vi "TempControllerMain.vi"() -> ()   [LabVIEW 2013]
uses:
  Controls/stateEnum.ctl
panel:
  in  "Log Folder Location":path=path "E:/USB/LabView/TemperatureController/Data"
  out "Temperature (K)":dbl(graph)
  out "Current Temperature (simulated)":dbl
  out "Current Task":T1
  out "Current Temperature (real)":dbl
  out "Heating up":bool
  in  "Set Point (Max)":dbl
  in  "Monitor\nTemp":bool
  in  "Mode":bool
  in  "Calibrate":bool
  out "Room Temperature (K)":dbl
  out "Resistance @ Room Temperature (ohms)":dbl
  in  "stop":bool
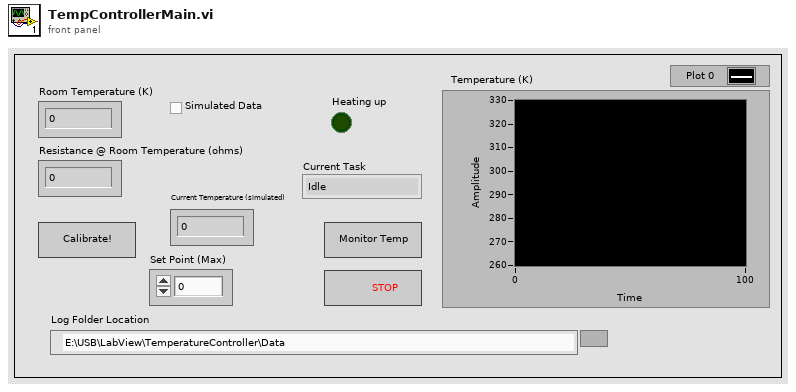
[diagram p1: front panel]
types:
  T1 = typedef "stateEnum.ctl" = enum16{"Idle", "Calibrate", "Initialise", "Set Voltage On", "Set Voltage Off", "Exit"}
  T2 = enum16{"open", "open or create", "create or replace", "create", "open (read-only)"}
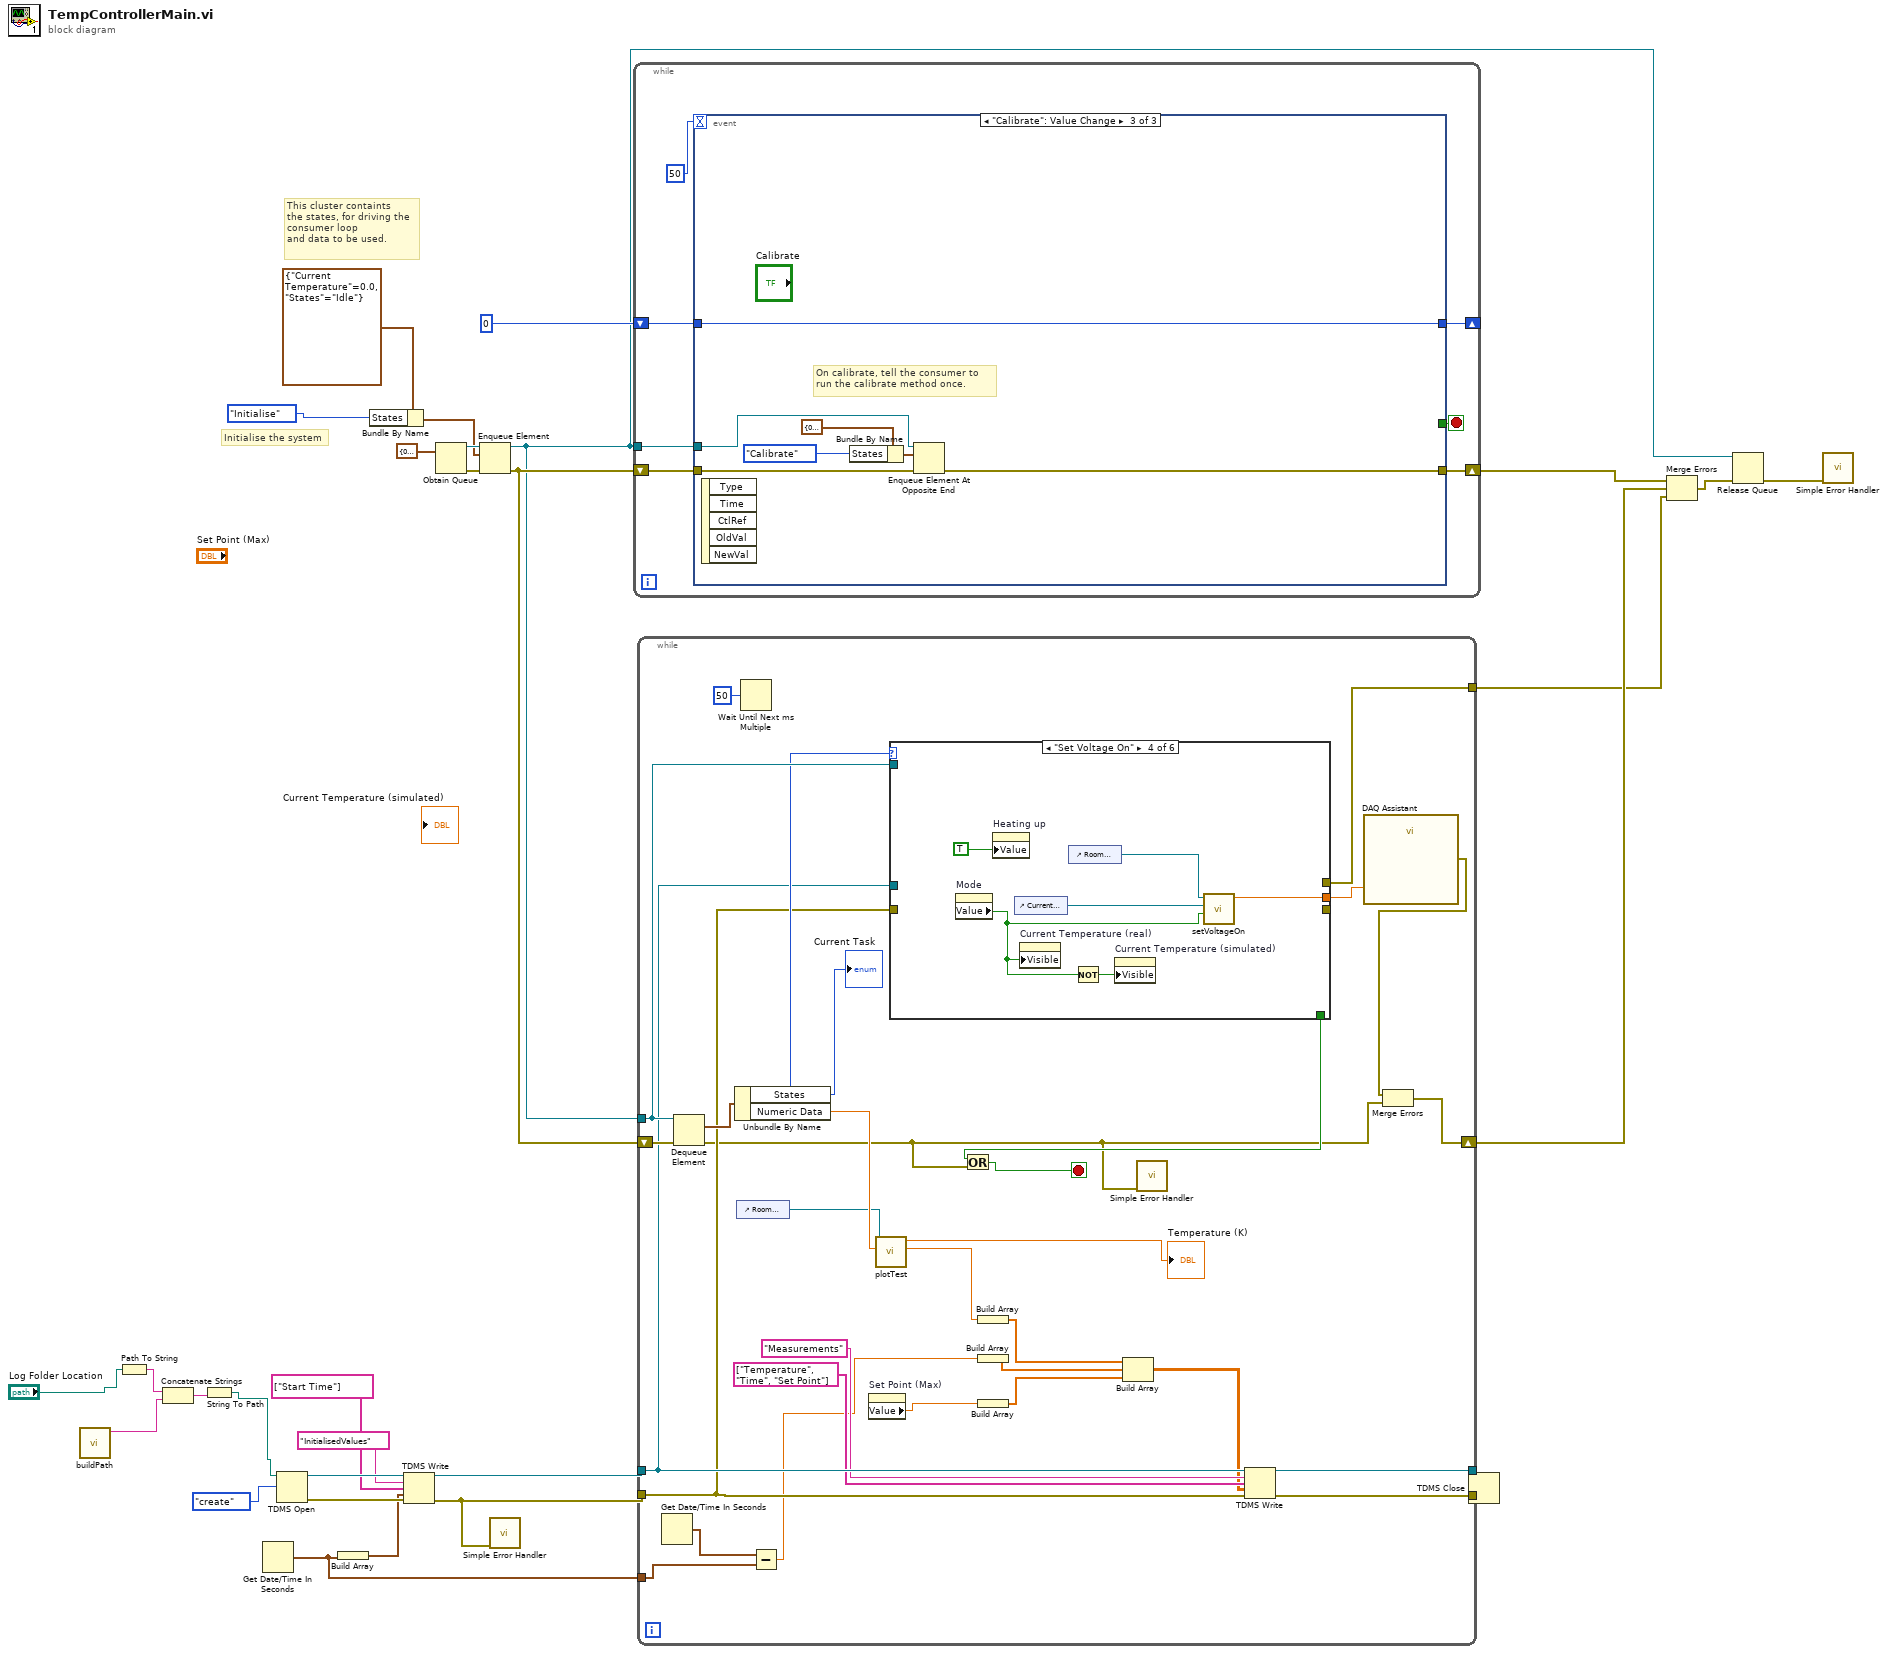
[diagram p0: block diagram]
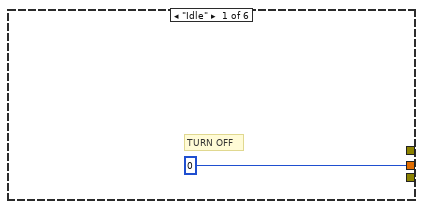
[diagram p2: hidden frame]
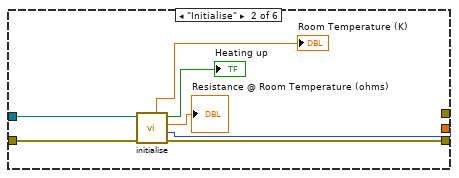
[diagram p3: hidden frame]
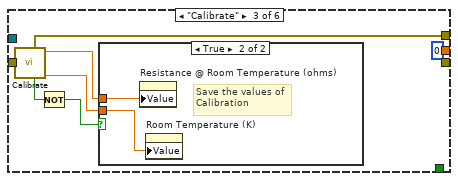
[diagram p4: hidden frame]
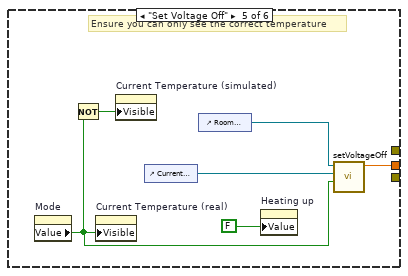
[diagram p6: hidden frame]
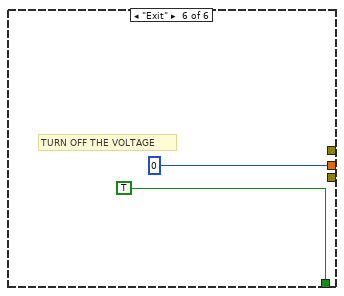
[diagram p7: hidden frame]
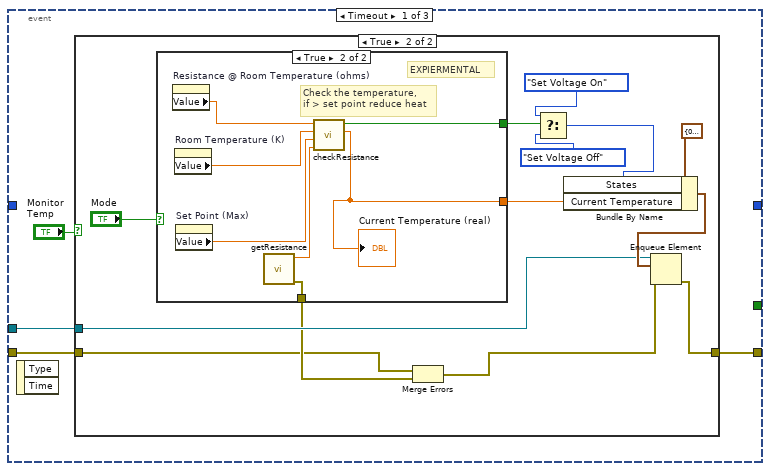
[diagram p8: hidden frame]
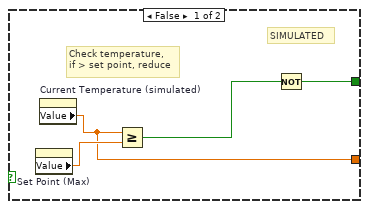
[diagram p10: hidden frame]
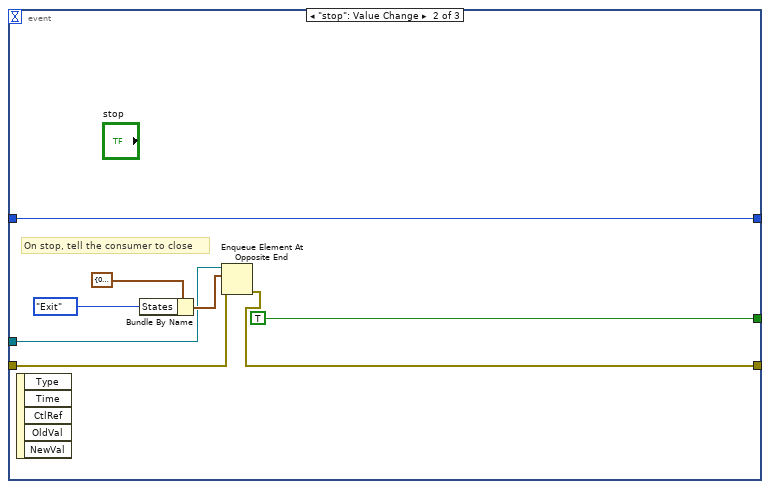
[diagram p11: hidden frame]
diagram:
  # "Initialise the system"
  # "This cluster containts\nthe states, for driving the\nconsumer loop\nand data to be used."
  n1 = call "buildPath.vi"() -> ("String"=w3:string)  [unwired: 11 in]
  n2 = Path To String(path="Log Folder Location") -> (string=w4:string)
  n3 = Concatenate Strings(w4, w3) -> (w2:string)
  n4 = String To Path(string=w2) -> (path=w1:path)
  n5 = Get Date/Time In Seconds() -> (seconds since 1Jan1904=w7:timestamp)
  n6 = TDMS Open(10:T2."create" ("operation (0:open)"), 11:w1) -> (0:w11:errorcluster, 3:w13:refnum<k34>)  [unwired: 5 in]
  n7 = Build Array(w7) -> (w8:timestamp[])
  n8 = Bundle By Name(cluster=cluster{"Current Temperature":dbl, "States":T1} {"Current Temperature"=0.0, "States"=enum."Idle"}, "States"=stateEnum."Initialise") -> (w25:cluster{"Current Temperature":dbl, "States":T1})
  n9 = TDMS Write(0:w13, 5:"InitialisedValues" ("group name in (Untitled)"), 7:string[] ["Start Time"] ("channel name(s) in (Untitled)"), 9:w8, 11:w11) -> (4:w12:refnum<k34>, 15:w6:errorcluster)  [unwired: 1 in, 2 out]
  n10 = Obtain Queue(element data type=cluster{"Numeric Data":dbl, "States":T1} {"Numeric Data"=0.0, "States"=enum."Idle"}) -> (queue out=w29:refnum<queue>, error out=w28:errorcluster)  [unwired: 4 in, 1 out]
  n11 = Enqueue Element(queue=w29, element=w25, error in (no error)=w28) -> (queue out=w19:refnum<queue>, error out=w27:errorcluster)  [unwired: 1 in, 1 out]
  n12 = call <vilib>:"Simple Error Handler.vi"("error in (no error)"=w6) -> ()  [unwired: 4 in, 5 out]
  n13 = while {
    tunnel: w19 -> [w37]
    shift-right: [w34] -> w21
    shift-left: w27 -> [w36]
    shift-right: [w31] -> _
    shift-left: 0 -> [w32]
    stop <- w35 stop-if-true
    n14 = event shown="[2] \"Calibrate\": Value Change" {
      selector: _ -> [_ _ _]
      dyn-events: _ -> [_ _ _]
      timeout: 50 -> [_ _ _]
      tunnel: w37 -> [w41 w69 w80]
      tunnel: w36 -> [w40 w68 w79]
      tunnel: [w38 w67 w78] -> w34
      tunnel: [_ TRUE _] -> w35
      tunnel: w32 -> [_ w73 w75]
      tunnel: [_ w73 w75] -> w31
      event Timeout {
        n15 = event-data() -> ()  [unwired: 1 in, 2 out]
        n16 = case shown="True" "Monitor\nTemp" {
          tunnel: w41 -> [_ w53]
          tunnel: w40 -> [w42 w45]
          tunnel: [w42 w43] -> w38
          frame False {
          }
          frame True {
            n17 = case shown="True" "Mode" {
              tunnel: [w58 w62] -> w52
              tunnel: [w56 w61] -> w50
              tunnel: [_ w60] -> w46
              frame False {
                # "SIMULATED"
                # "Check temperature,\nif > set point, reduce"
                n18 = property on="Set Point (Max)" class="DigNum (strict)"() -> ("Value"=w59:dbl)  [unwired: 2 in, 2 out]
                n19 = property on="Current Temperature (simulated)" class="DigNum (strict)"() -> ("Value"=w58:dbl)  [unwired: 2 in, 2 out]
                n20 = Greater Or Equal?(x=w58, y=w59) -> (x >= y?=w57:bool)
                n21 = Not(x=w57) -> (.not. x?=w56:bool)
              }
              frame True {
                # "EXPIERMENTAL"
                # "Check the temperature, \nif > set point reduce heat"
                n22 = property on="Resistance @ Room Temperature (ohms)" class="DigNum (strict)"() -> ("Value"=w66:dbl)  [unwired: 2 in, 2 out]
                n23 = property on="Room Temperature (K)" class="DigNum (strict)"() -> ("Value"=w65:dbl)  [unwired: 2 in, 2 out]
                n24 = property on="Set Point (Max)" class="DigNum (strict)"() -> ("Value"=w64:dbl)  [unwired: 2 in, 2 out]
                n25 = call "getResistance.vi"() -> ("error out"=w60:errorcluster, "Resistance (ohms)"=w63:dbl)  [unwired: 9 in, 1 out]
                n26 = call "checkResistance.vi"("Current Resistance"=w63, "Set Temperature"=w64, "Calibrated Temperature"=w65, "Calibrated Resistance"=w66) -> ("Current Temperature"=w62:dbl, "Turn Voltage On?"=w61:bool)  [unwired: 6 in]
                "Current Temperature (real)" <- w62
              }
            }
            n27 = Merge Errors(w45, w46) -> (w44:errorcluster)
            n28 = Select(t=stateEnum."Set Voltage On" ("States"), s=w50, f=stateEnum."Set Voltage Off" ("States")) -> (s? t:f=w47:T1)
            n29 = Bundle By Name(cluster=cluster{"Current Temperature":dbl, "States":T1} {"Current Temperature"=0.0, "States"=enum."Idle"}, "States"=w47, "Current Temperature"=w52) -> (w54:cluster{"Current Temperature":dbl, "States":T1})
            n30 = Enqueue Element(queue=w53, element=w54, error in (no error)=w44) -> (error out=w43:errorcluster)  [unwired: 1 in, 2 out]
          }
        }
      }
      event "stop": Value Change {
        # "On stop, tell the consumer to close"
        n31 = event-data() -> ()  [unwired: 1 in, 5 out]
        n32 = Bundle By Name(cluster=cluster{"Current Temperature":dbl, "States":T1} {"Current Temperature"=0.0, "States"=enum."Idle"}, "States"=stateEnum."Exit") -> (w70:cluster{"Current Temperature":dbl, "States":T1})
        n33 = Enqueue Element At Opposite End(queue=w69, element=w70, error in (no error)=w68) -> (error out=w67:errorcluster)  [unwired: 1 in, 2 out]
      }
      event "Calibrate": Value Change {
        # "On calibrate, tell the consumer to \nrun the calibrate method once."
        n34 = event-data() -> ()  [unwired: 1 in, 5 out]
        n35 = Bundle By Name(cluster=cluster{"Current Temperature":dbl, "States":T1} {"Current Temperature"=0.0, "States"=enum."Idle"}, "States"=stateEnum."Calibrate") -> (w76:cluster{"Current Temperature":dbl, "States":T1})
        n36 = Enqueue Element At Opposite End(queue=w80, element=w76, error in (no error)=w79) -> (error out=w78:errorcluster)  [unwired: 1 in, 2 out]
      }
    }
  }
  n37 = while {
    shift-right: [w84] -> w22
    shift-left: w27 -> [w111]
    tunnel: w19 -> [w108]
    tunnel: [w102] -> w18
    tunnel: w12 -> [w101]
    tunnel: w6 -> [w100]
    tunnel: [w92] -> w15
    tunnel: [w91] -> w14
    tunnel: w7 -> [w89]
    stop <- w106 stop-if-true
    n38 = Get Date/Time In Seconds() -> (seconds since 1Jan1904=w90:timestamp)
    n39 = Dequeue Element(queue=w108, error in (no error)=w111) -> (element=w110:cluster{"Numeric Data":dbl, "States":T1}, error out=w85:errorcluster)  [unwired: 1 in, 2 out]
    n40 = Unbundle By Name(w110) -> ("States"=w105:T1, "Numeric Data"=w104:dbl)
    "Current Task" <- w105
    n41 = control-ref of="Room Temperature (K)"() -> (w83:refnum<vi>)
    n42 = Wait Until Next ms Multiple(millisecond multiple=u32 50) -> ()  [unwired: 1 out]
    n43 = Subtract(x=w90, y=w89) -> (x-y=w88:dbl)
    n44 = property on="Set Point (Max)" class="DigNum (strict)"() -> ("Value"=w96:dbl)  [unwired: 2 in, 2 out]
    n45 = call "plotTest.vi"("Current Temp"=w104, "Room Temperure (K)"=w83) -> ("Current Temperature"=w97:dbl, "Temperature (K)"=→"Temperature (K)":dbl)  [unwired: 8 in]
    n46 = case shown="\"Set Voltage On\"" w105 {
      tunnel: w108 -> [_ _ _ _ _ _]
      tunnel: [_ _ _ _ _ TRUE] -> w107
      tunnel: [0 w119 0 w130 w136 0] -> w103
      tunnel: [_ _ w120 _ _ _] -> w102
      tunnel: w101 -> [_ w117 _ _ _ _]
      tunnel: w100 -> [_ w118 _ _ _ _]
      tunnel: [_ w116 _ _ _ _] -> _
      frame "Idle" {
        # "TURN OFF"
      }
      frame "Initialise" {
        n47 = call "initialise.vi"("error in (no error)"=w118, "Refnum in"=w117) -> ("error out"=w116:errorcluster, "Numeric Control"=w119:i32, "Resistance @ Room Temperature (ohms)"=→"Resistance @ Room Temperature (ohms)":dbl, "Heating up"=→"Heating up":bool, "Room Temperature (K)"=→"Room Temperature (K)":dbl)  [unwired: 5 in]
      }
      frame "Calibrate" {
        n48 = call "Calibrate.vi"() -> ("Calib Temperature"=w124:dbl, "Calibration Resistance (ohms)"=w125:dbl, "Canceled"=w122:bool, "error out"=w120:errorcluster)  [unwired: 6 in, 2 out]
        n49 = Not(x=w122) -> (.not. x?=w123:bool)
        n50 = case shown="True" w123 {
          tunnel: w125 -> [_ w127]
          tunnel: w124 -> [_ w126]
          frame False {
            # "If you cancel the calibration\ndon't save the values!"
          }
          frame True {
            # "Save the values of\nCalibration"
            n51 = property on="Resistance @ Room Temperature (ohms)" class="DigNum (strict)"("Value"=w127) -> ()  [unwired: 2 in, 2 out]
            n52 = property on="Room Temperature (K)" class="DigNum (strict)"("Value"=w126) -> ()  [unwired: 2 in, 2 out]
          }
        }
      }
      frame "Set Voltage On" {
        n53 = property on="Mode" class="Bool (strict)"() -> ("Value"=w131:bool)  [unwired: 2 in, 2 out]
        n54 = property on="Heating up" class="Bool (strict)"("Value"=TRUE ("Voltage")) -> ()  [unwired: 2 in, 2 out]
        n55 = control-ref of="Current Temperature (simulated)"() -> (w128:refnum<vi>)
        n56 = property on="Current Temperature (real)" class="DigNum (strict)"("Visible"=w131) -> ()  [unwired: 2 in, 2 out]
        n57 = control-ref of="Room Temperature (K)"() -> (w129:refnum<vi>)
        n58 = Not(x=w131) -> (.not. x?=w132:bool)
        n59 = property on="Current Temperature (simulated)" class="DigNum (strict)"("Visible"=w132) -> ()  [unwired: 2 in, 2 out]
        n60 = call "setVoltageOn.vi"("Mode"=w131, "Current Temperature (Simulated)"=w128, "Room Temperature (K)"=w129) -> ("Value"=w130:dbl)  [unwired: 8 in]
      }
      frame "Set Voltage Off" {
        # "Ensure you can only see the correct temperature"
        n61 = property on="Mode" class="Bool (strict)"() -> ("Value"=w138:bool)  [unwired: 2 in, 2 out]
        n62 = Not(x=w138) -> (.not. x?=w137:bool)
        n63 = property on="Current Temperature (real)" class="DigNum (strict)"("Visible"=w138) -> ()  [unwired: 2 in, 2 out]
        n64 = property on="Current Temperature (simulated)" class="DigNum (strict)"("Visible"=w137) -> ()  [unwired: 2 in, 2 out]
        n65 = control-ref of="Current Temperature (simulated)"() -> (w134:refnum<vi>)
        n66 = control-ref of="Room Temperature (K)"() -> (w135:refnum<vi>)
        n67 = property on="Heating up" class="Bool (strict)"("Value"=FALSE ("Voltage")) -> ()  [unwired: 2 in, 2 out]
        n68 = call "setVoltageOff.vi"("Mode"=w138, "Current Temperature (simulated)"=w134, "Room Temperature (K)"=w135) -> ("Voltage"=w136:dbl)  [unwired: 8 in]
      }
      frame "Exit" {
        # "TURN OFF THE VOLTAGE"
      }
    }
    n69 = Or(x=w107, y=w85) -> (x .or. y?=w106:bool)
    n70 = Build Array(w97) -> (w95:dbl[])
    n71 = Build Array(w88) -> (w87:dbl[])
    n72 = Build Array(w96) -> (w94:dbl[])
    n73 = Build Array(w95, w87, w94) -> (w93:dbl[][])
    n74 = call <vilib>:"Simple Error Handler.vi"("error in (no error)"=w85) -> ()  [unwired: 4 in, 5 out]
    n75 = TDMS Write(0:w101, 5:"Measurements" ("group name in (Untitled)"), 7:string[] ["Temperature", "Time", "Set Point"], 9:w93, 11:w100) -> (4:w92:refnum<k34>, 15:w91:errorcluster)  [unwired: 1 in, 2 out]
    n76 = call "DAQ Assistant"("data"=w103) -> ("error out"=w86:errorcluster)  [unwired: 17 in, 1 out]
    n77 = Merge Errors(w86, w85) -> (w84:errorcluster)
  }
  n78 = TDMS Close(8:w14, 11:w15) -> ()  [unwired: 2 out]
  n79 = Merge Errors(w21, w22, w18) -> (w20:errorcluster)
  n80 = Release Queue(queue=w19, error in (no error)=w20) -> (error out=w17:errorcluster)  [unwired: 1 in, 2 out]
  n81 = call <vilib>:"Simple Error Handler.vi"("error in (no error)"=w17) -> ()  [unwired: 4 in, 5 out]
